vi "FTW-Supervisor-Shutdown.vi"(0 "FTW Supervisor Connection":T1, 11 "error in":errorcluster) -> (15 "error out":errorcluster)   [LabVIEW 2015]
uses:
  core/type/FTW-Type-Actor-Connector.ctl
panel:
  in  "Timeout":i32=5000 format="%dmsec"
  # "Inputs"
  # "Outputs"
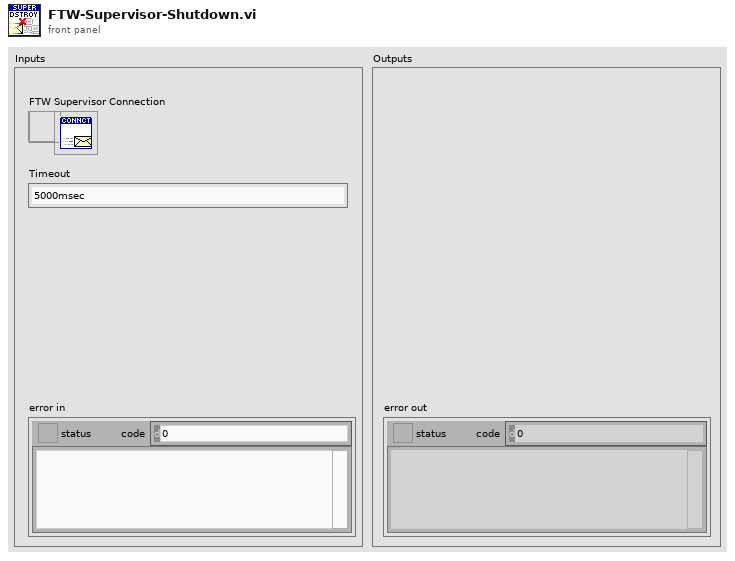
[diagram p1: front panel]
types:
  T1 = typedef "FTW-Type-Actor-Connector.ctl" = refnum<data-value>
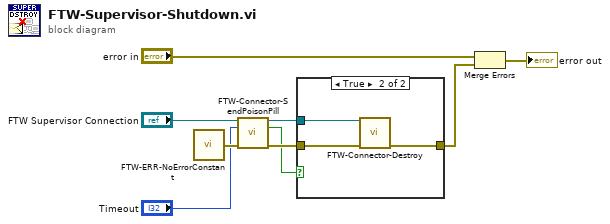
[diagram p0: block diagram]
diagram:
  n1 = call "FTW-ERR-NoErrorConstant.vi"() -> ("no error"=w4:errorcluster)
  n2 = call "FTW-Connector-SendPoisonPill.vi"("FTW Actor Connector"="FTW Supervisor Connection", "Timeout"="Timeout", "error in"=w4) -> ("FTW Actor Connector out"=w7:T1, "Shutting Down?"=w2:bool, "error out"=w6:errorcluster)  [unwired: 9 in, 1 out]
  n3 = case shown="True" w2 {
    tunnel: w7 -> [_ w13]
    tunnel: w6 -> [w10 w12]
    tunnel: [w10 w11] -> w5
    frame False {
    }
    frame True {
      n4 = call "FTW-Connector-Destroy.vi"("FTW Actor Connector"=w13, "error in"=w12) -> ("error out"=w11:errorcluster)  [unwired: 13 in]
    }
  }
  n5 = Merge Errors("error in", w5) -> (→"error out":errorcluster)
